vi "Periodic Tasks.vi"() -> ()   [LabVIEW 2011]
doc: "This VI runs in parallel to other tasks. It can contain as many user-defined periodic loops as you need. These can carry out PID or other sorts of timed response."
uses:
  <vilib>/Rock Robotics/SystemInterfaces/Utilities/FPGA_UtilitiesLED State.ctl
  <vilib>/Rock Robotics/SystemInterfaces/Utilities/FPGA_UtilitiesLED Source.ctl
  <vilib>/Rock Robotics/WPI/Relay/WPI_RelayValue.ctl
  Robot Global Data.vi
panel:
  out "Sent?":string="File Wrote"
  out "Voltage":dbl
  in  "Recording Array":dbl[][](array[numeric])
  in  "Turn on Record 2":bool
  out "Auton Recording 2":bool
  in  "Home Speed 2":dbl=1.0
  out "Ramp ACT Pot 2":dbl
  out "Auton Recording":bool
  in  "Turn on Record":bool
  in  "Auton Array":dbl[][](array[numeric])
  out "Right Rate":dbl
  out "Right Direction":bool
  out "Right Distance":dbl
  out "Shooter Encoder Distance":dbl
  out "Shooter Direction":bool
  out "Shooter Encoder Rate":dbl
  out "Left Rate":dbl
  out "Gyro Rate":dbl
  out "Gyro Angle":dbl
  out "Left Direction":bool
  out "Left Distance":dbl
  # "Auton Recording"
  # "Sensor Feedback"
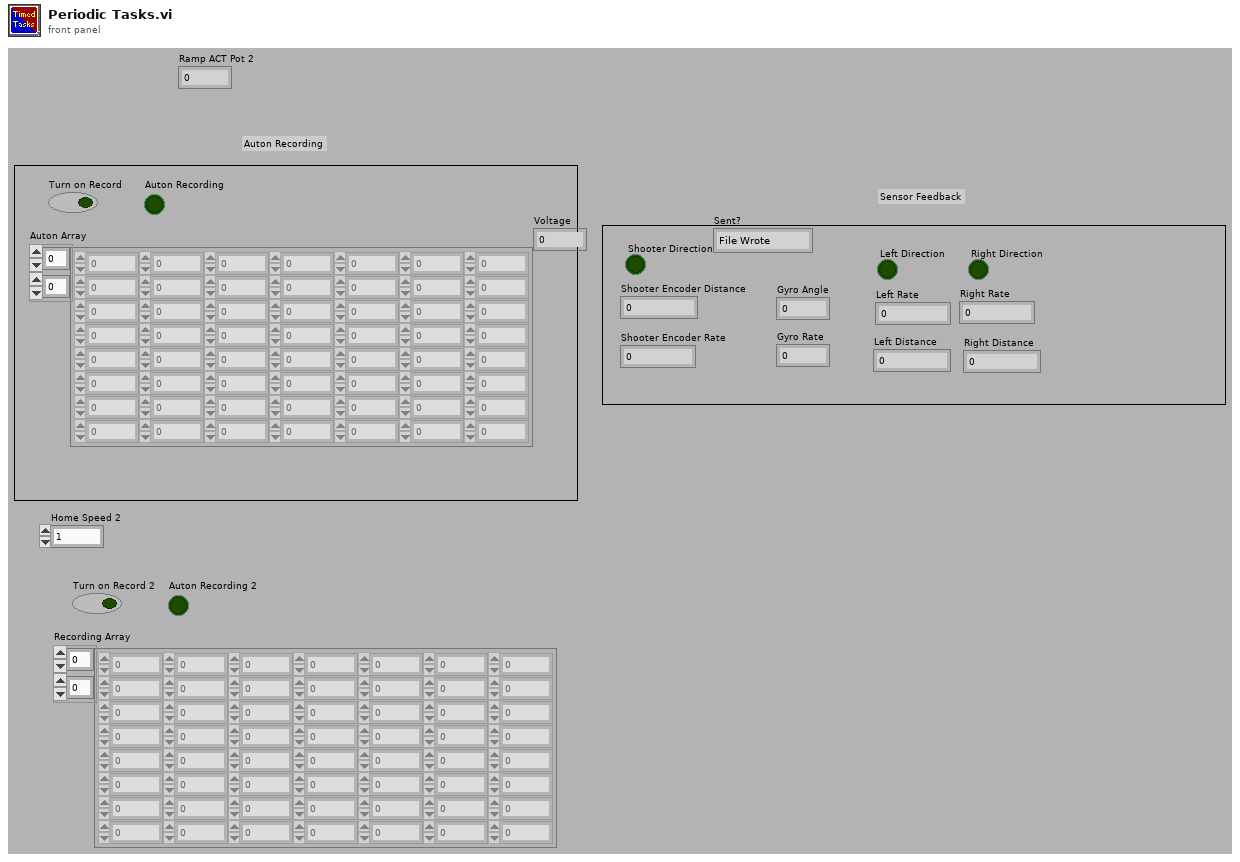
[diagram p1: front panel]
types:
  T1 = typedef "WPI_RelayValue.ctl" = enum16{"Off", "On", "Forward", "Reverse"}
  T2 = cluster{"Driver Station Digital Input (1-8)[0]":bool, "Driver Station Digital Input (1-8)[1]":bool, "Driver Station Digital Input (1-8)[2]":bool, "Driver Station Digital Input (1-8)[3]":bool, "Driver Station Digital Input (1-8)[4]":bool, "Driver Station Digital Input (1-8)[5]":bool, "Driver Station Digital Input (1-8)[6]":bool, "Driver Station Digital Input (1-8)[7]":bool, "Driver Station Digital Input (1-8)[8]":bool}
  T3 = typedef "WPI_AnalogChannelDevRef.ctl" = cluster{"DevStatus":errorcluster, "Analog Module":T4, "Analog Channel":T5}
  T4 = typedef "FPGA_TypedefAnalogModule.ctl" = enum16{"Analog Module 1", "Analog Module 2"}
  T5 = typedef "FPGA_AIChannel.ctl" = enum8{"AI 1", "AI 2", "AI 3", "AI 4", "AI 5", "AI 6", "AI 7", "AI 8", "Invalid"}
  T6 = typedef "WPI_EncoderDevRef.ctl" = cluster{"DevStatus":errorcluster, "EncoderIndex":T7, "CounterIndex":T8, "DistancePerCount":dbl, "Decoding Type":T9}
  T7 = typedef "FPGA_EncoderIdx.ctl" = enum8{"Enc 0", "Enc 1", "Enc 2", "Enc 3", "Invalid"}
  T8 = typedef "FPGA_CounterCtrSystemIndex.ctl" = enum8{"Ctr 0", "Ctr 1", "Ctr 2", "Ctr 3", "Ctr 4", "Ctr 5", "Ctr 6", "Ctr 7", "Invalid"}
  T9 = typedef "WPI_EncoderType.ctl" = enum16{"1x", "2x", "4x"}
  T10 = typedef "WPI_GyroDevRef.ctl" = cluster{"DevStatus":errorcluster, "Analog Module":T4, "Analog Channel":T5, "Offset":dbl, "Gain (VoltsPerDegree/Second)":dbl}
  T11 = typedef "WPI_RelayDevRef.ctl" = cluster{"DevStatus":errorcluster, "Relay Channel":T12, "Digital Module":T13, "Relay Direction":T14}
  T12 = typedef "FPGA_DIORelayChannel.ctl" = enum8{"Relay 1", "Relay 2", "Relay 3", "Relay 4", "Relay 5", "Relay 6", "Relay 7", "Relay 8", "Invalid"}
  T13 = typedef "FPGA_TypedefDigitalModule.ctl" = enum16{"Digital Module 1", "Digital Module 2"}
  T14 = typedef "WPI_RelayDirection.ctl" = enum16{"Both directions", "Forward only", "Reverse only"}
  T15 = typedef "FPGA_UtilitiesLED State.ctl" = enum16{"Off", "On", "Toggle"}
  T16 = typedef "FPGA_UtilitiesLED Source.ctl" = enum16{"User LED", "FPGA LED"}
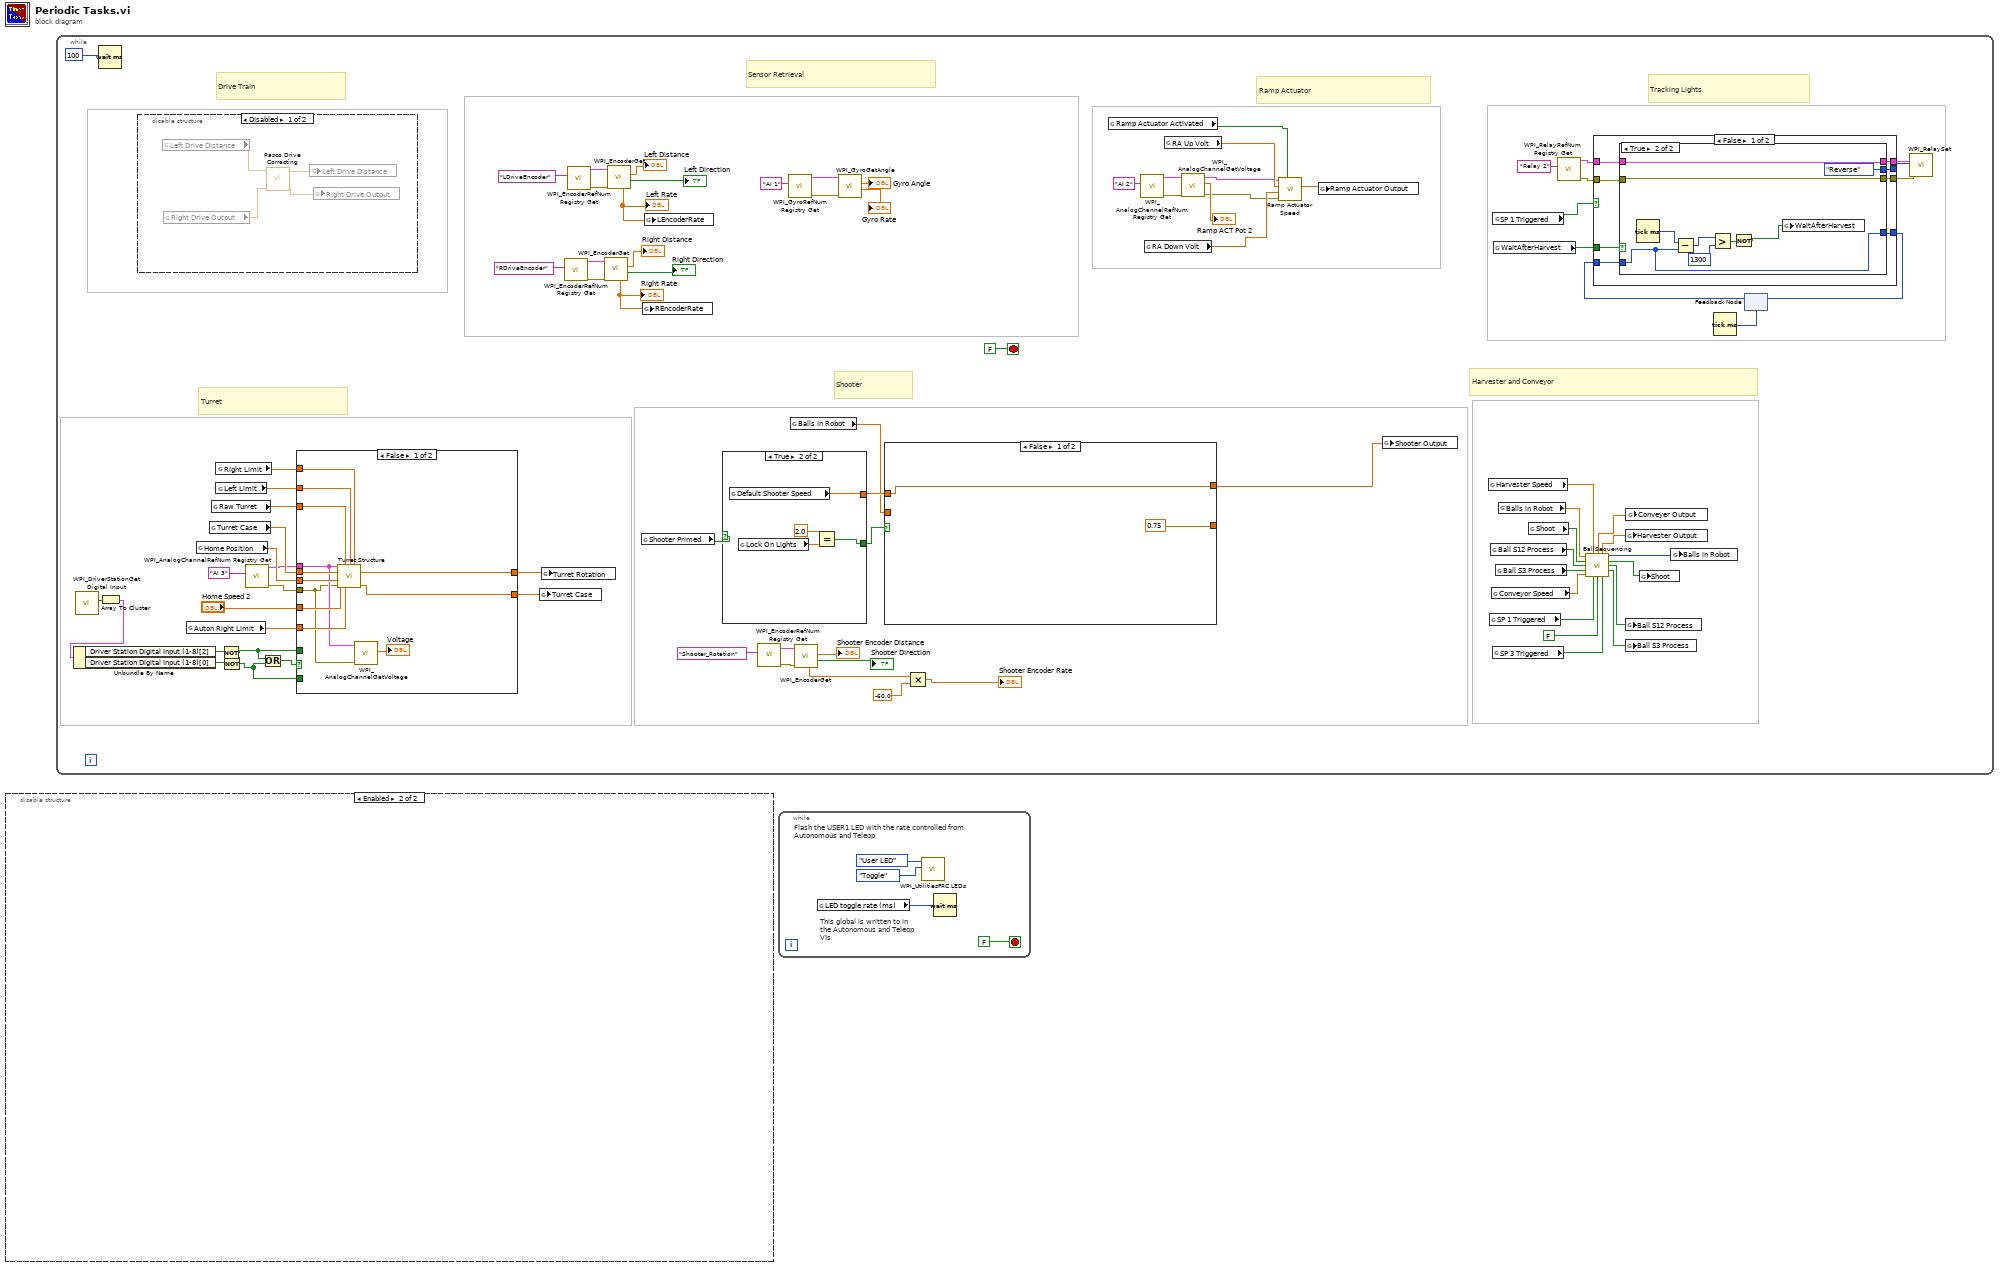
[diagram p0: block diagram]
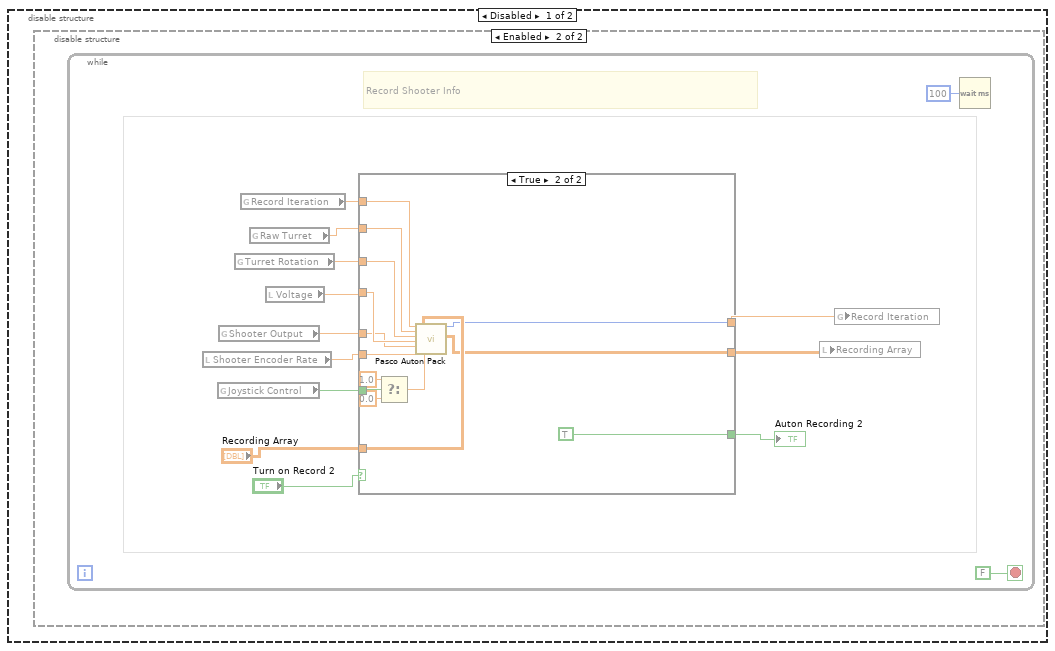
[diagram p2: hidden frame]
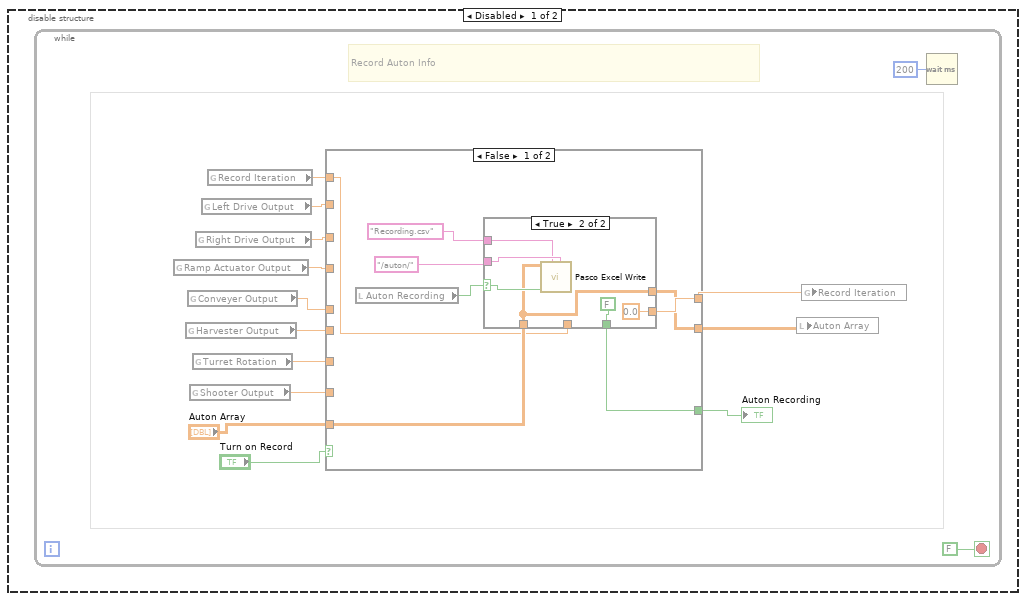
[diagram p3: hidden frame]
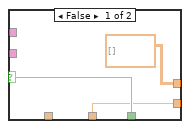
[diagram p4: hidden frame]
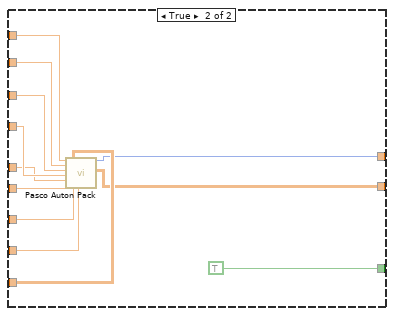
[diagram p5: hidden frame]
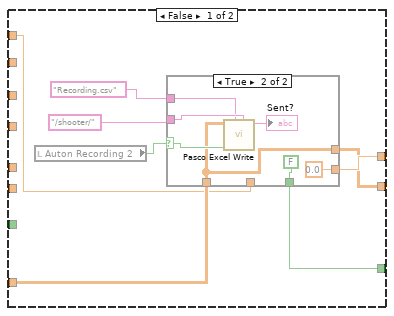
[diagram p6: hidden frame]
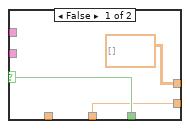
[diagram p7: hidden frame]
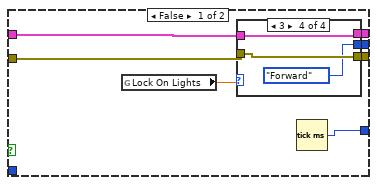
[diagram p8: hidden frame]
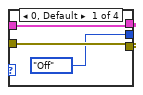
[diagram p9: hidden frame]
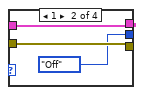
[diagram p10: hidden frame]
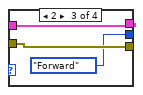
[diagram p11: hidden frame]
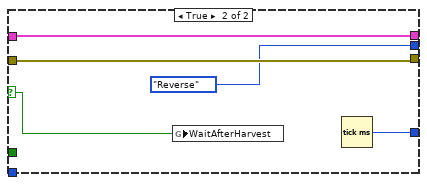
[diagram p12: hidden frame]
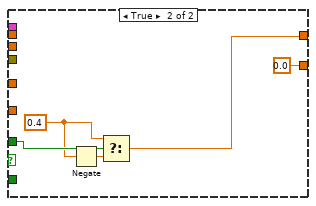
[diagram p13: hidden frame]
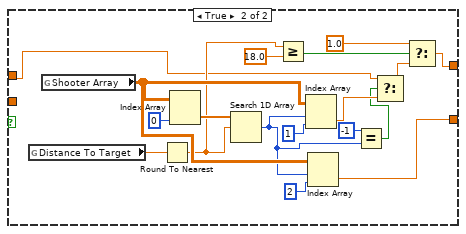
[diagram p14: hidden frame]
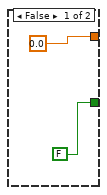
[diagram p15: hidden frame]
diagram:
  n1 = disable-structure shown="Enabled" {
    frame Disabled {
      n2 = disable-structure shown="Enabled" {
        frame Disabled {
          n3 = while {
            stop <- FALSE stop-if-true
            # "Record Auton Info"
            n4 = global read "Robot Global Data.vi" "Ramp Actuator Output"() -> (w5:dbl)
            n5 = global read "Robot Global Data.vi" "Harvester Output"() -> (w7:dbl)
            n6 = global read "Robot Global Data.vi" "Conveyer Output"() -> (w6:dbl)
            n7 = global read "Robot Global Data.vi" "Shooter Output"() -> (w9:dbl)
            n8 = global read "Robot Global Data.vi" "Turret Rotation"() -> (w8:dbl)
            n9 = global read "Robot Global Data.vi" "Right Drive Output"() -> (w4:dbl)
            n10 = global read "Robot Global Data.vi" "Left Drive Output"() -> (w3:dbl)
            n11 = global read "Robot Global Data.vi" "Record Iteration"() -> (w2:dbl)
            n12 = case shown="False" "Turn on Record" {
              tunnel: w2 -> [w19 w44]
              tunnel: w3 -> [_ w43]
              tunnel: w4 -> [_ w42]
              tunnel: w5 -> [_ w41]
              tunnel: w6 -> [_ w40]
              tunnel: w7 -> [_ w39]
              tunnel: w8 -> [_ w38]
              tunnel: w9 -> [_ w37]
              tunnel: "Auton Array" -> [w20 w36]
              tunnel: [w16 w35] -> w12
              tunnel: [w17 w34] -> w13
              tunnel: [w18 TRUE] -> w14
              frame False {
                n13 = local read "Auton Recording"() -> (w21:bool)
                n14 = case shown="True" w21 {
                  selector: w21 -> [w26 w31]
                  tunnel: [w26 FALSE] -> w18
                  tunnel: "/auton/" ("File Name") -> [_ w30]
                  tunnel: "Recording.csv" ("Folder Location") -> [_ w29]
                  tunnel: [w25 0.0 ("Record Iteration")] -> w17
                  tunnel: w19 -> [w25 _]
                  tunnel: w20 -> [_ w27]
                  tunnel: [dbl[][] [] ("Auton Array") w27] -> w16
                  frame False {
                  }
                  frame True {
                    n15 = call "Pasco Excel Write.vi"("Folder Location"=w30, "File Name"=w29, "WriteToExcel"=w31, "2D data"=w27) -> ()  [unwired: 7 in, 1 out]
                  }
                }
              }
              frame True {
                n16 = call "Pasco Auton Pack.vi"("Iterations"=w44, "Left Drive"=w43, "Right Drive"=w42, "RAMP ACT"=w41, "Conveyor"=w40, "Harvestor"=w39, "Auton Array"=w36, "Turret"=w38, "Shooter"=w37) -> ("Iteration Output"=w34:i32, "output array"=w35:dbl[][])  [unwired: 9 in]
              }
            }
            "Auton Recording" <- w14
            n17 = local write "Auton Array"(w12) -> ()
            n18 = global write "Robot Global Data.vi" "Record Iteration"(w13) -> ()
            n19 = Wait (ms)(milliseconds to wait=u32 200) -> ()  [unwired: 1 out]
          }
        }
        frame Enabled {
          n20 = while {
            stop <- FALSE stop-if-true
            # "Record Shooter Info"
            n21 = local read "Shooter Encoder Rate"() -> (w46:dbl)
            n22 = global read "Robot Global Data.vi" "Joystick Control"() -> (w45:bool)
            n23 = global read "Robot Global Data.vi" "Shooter Output"() -> (w47:dbl)
            n24 = global read "Robot Global Data.vi" "Turret Rotation"() -> (w49:dbl)
            n25 = global read "Robot Global Data.vi" "Record Iteration"() -> (w52:dbl)
            n26 = global read "Robot Global Data.vi" "Raw Turret"() -> (w50:dbl)
            n27 = local read "Voltage"() -> (w48:dbl)
            n28 = case shown="True" "Turn on Record 2" {
              tunnel: w52 -> [w62 w90]
              tunnel: w50 -> [_ w89]
              tunnel: w49 -> [_ w88]
              tunnel: w48 -> [_ w87]
              tunnel: w47 -> [_ w86]
              tunnel: w46 -> [_ w85]
              tunnel: "Recording Array" -> [w63 w84]
              tunnel: [w59 w83] -> w55
              tunnel: [w60 w82] -> w56
              tunnel: [w61 TRUE] -> w57
              tunnel: w45 -> [_ w80]
              frame False {
                n29 = local read "Auton Recording 2"() -> (w64:bool)
                n30 = case shown="True" w64 {
                  selector: w64 -> [w69 w75]
                  tunnel: [w69 FALSE] -> w61
                  tunnel: "/shooter/" ("File Name") -> [_ w74]
                  tunnel: "Recording.csv" ("Folder Location") -> [_ w73]
                  tunnel: [w68 0.0 ("Record Iteration")] -> w60
                  tunnel: w62 -> [w68 _]
                  tunnel: w63 -> [_ w71]
                  tunnel: [dbl[][] [] ("Auton Array") w71] -> w59
                  frame False {
                  }
                  frame True {
                    n31 = call "Pasco Excel Write.vi"("Folder Location"=w74, "File Name"=w73, "WriteToExcel"=w75, "2D data"=w71) -> ("Sent?"=→"Sent?":string)  [unwired: 7 in]
                  }
                }
              }
              frame True {
                n32 = Select(t=1.0, s=w80, f=0.0) -> (s? t:f=w77:dbl)
                n33 = call "Pasco Auton Pack.vi"("Iterations"=w90, "Left Drive"=w89, "Right Drive"=w88, "RAMP ACT"=w87, "Conveyor"=w86, "Harvestor"=w85, "Auton Array"=w84, "Turret"=w77) -> ("Iteration Output"=w82:i32, "output array"=w83:dbl[][])  [unwired: 10 in]
              }
            }
            "Auton Recording 2" <- w57
            n34 = local write "Recording Array"(w55) -> ()
            n35 = global write "Robot Global Data.vi" "Record Iteration"(w56) -> ()
            n36 = Wait (ms)(milliseconds to wait=u32 100) -> ()  [unwired: 1 out]
          }
        }
      }
    }
    frame Enabled {
    }
  }
  n37 = while {
    stop <- FALSE stop-if-true
    # "Tracking Lights"
    # "Harvester and Conveyor"
    # "Shooter"
    # "Sensor Retrieval"
    # "Turret"
    # "Drive Train"
    # "Ramp Actuator"
    n38 = call <vilib>:"WPI_DriverStationGet Digital Input.vi"() -> ("Driver Station Digital Input (1-8)"=w120:bool[])  [unwired: 11 in]
    n39 = Wait (ms)(milliseconds to wait=u32 100) -> ()  [unwired: 1 out]
    n40 = Array To Cluster(array=w120) -> (cluster=w119:T2)
    n41 = Unbundle By Name(w119) -> ("Driver Station Digital Input (1-8)[2]"=w105:bool, "Driver Station Digital Input (1-8)[0]"=w103:bool)
    n42 = disable-structure shown="Disabled" {
      frame Disabled {
        n43 = global read "Robot Global Data.vi" "Left Drive Distance"() -> (w265:dbl)
        n44 = global read "Robot Global Data.vi" "Right Drive Output"() -> (w264:dbl)
        n45 = call "Pasco Drive Correcting.vi"("RightDriveOutput"=w264, "LeftDriveOutput"=w265) -> ("RightDriveOutput"=w262:dbl, "LeftDriveOutput"=w263:dbl)  [unwired: 8 in]
        n46 = global write "Robot Global Data.vi" "Left Drive Distance"(w263) -> ()
        n47 = global write "Robot Global Data.vi" "Right Drive Output"(w262) -> ()
      }
      frame Enabled {
      }
    }
    n48 = global read "Robot Global Data.vi" "Auton Right Limit"() -> (w116:dbl)
    n49 = global read "Robot Global Data.vi" "Home Position"() -> (w111:dbl)
    n50 = global read "Robot Global Data.vi" "Turret Case"() -> (w110:dbl)
    n51 = global read "Robot Global Data.vi" "Raw Turret"() -> (w112:dbl)
    n52 = global read "Robot Global Data.vi" "Right Limit"() -> (w115:dbl)
    n53 = global read "Robot Global Data.vi" "Left Limit"() -> (w114:dbl)
    n54 = Not(x=w105) -> (.not. x?=w104:bool)
    n55 = Not(x=w103) -> (.not. x?=w102:bool)
    n56 = call <vilib>:"WPI_AnalogChannelRefNum Registry Get.vi"("refnum name"="AI 3") -> ("error out"=w109:errorcluster, "AIDeviceRef"=w108:T3)  [unwired: 9 in]
    n57 = Or(x=w104, y=w102) -> (x .or. y?=w106:bool)
    n58 = case shown="False" w106 {
      tunnel: w108 -> [w221 _]
      tunnel: w109 -> [w220 _]
      tunnel: w110 -> [w230 _]
      tunnel: w111 -> [w229 _]
      tunnel: w112 -> [w228 _]
      tunnel: "Home Speed 2" -> [w227 _]
      tunnel: w114 -> [w226 _]
      tunnel: w115 -> [w225 _]
      tunnel: w116 -> [w224 _]
      tunnel: [w223 w234] -> w117
      tunnel: [w222 0.0 ("Turret Case Output")] -> w118
      tunnel: w104 -> [_ w235]
      tunnel: w102 -> [_ _]
      frame False {
        n59 = call "Turret Structure.vi"("AIDeviceRef"=w221, "Raw Turret"=w228, "Left"=w226, "Right"=w225, "Turret Case"=w230, "Home Speed"=w227, "Home postion"=w229, "error in (no error)"=w220, "Auton Right"=w224) -> ("Turret Output"=w223:dbl, "Turret Case Output"=w222:dbl)  [unwired: 5 in]
        n60 = call <vilib>:"WPI_AnalogChannelGetVoltage.vi"("error in (no error)"=w220, "AIDeviceRef"=w221) -> ("Voltage"=→"Voltage":dbl)  [unwired: 7 in, 2 out]
      }
      frame True {
        w231 = 0.4 ("t")
        n61 = Negate(x=w231) -> (-x=w232:dbl)
        n62 = Select(t=w231, s=w235, f=w232) -> (s? t:f=w234:dbl)
      }
    }
    n63 = global write "Robot Global Data.vi" "Turret Case"(w118) -> ()
    n64 = global write "Robot Global Data.vi" "Turret Rotation"(w117) -> ()
    n65 = call <vilib>:"WPI_EncoderRefNum Registry Get.vi"("refnum name"="RDriveEncoder") -> ("error out"=w144:errorcluster, "EncoderDevRef"=w143:T6)  [unwired: 9 in]
    n66 = call <vilib>:"WPI_EncoderRefNum Registry Get.vi"("refnum name"="LDriveEncoder") -> ("error out"=w150:errorcluster, "EncoderDevRef"=w149:T6)  [unwired: 9 in]
    n67 = call <vilib>:"WPI_EncoderGet.vi"("error in (no error)"=w144, "EncoderDevRef"=w143) -> ("Direction"=→"Right Direction":bool, "Distance"=→"Right Distance":dbl, "Rate"=w140:dbl)  [unwired: 4 in, 3 out]
    "Right Rate" <- w140
    n68 = call <vilib>:"WPI_EncoderGet.vi"("error in (no error)"=w150, "EncoderDevRef"=w149) -> ("Direction"=→"Left Direction":bool, "Distance"=→"Left Distance":dbl, "Rate"=w146:dbl)  [unwired: 4 in, 3 out]
    "Left Rate" <- w146
    n69 = global read "Robot Global Data.vi" "Shooter Primed"() -> (w164:bool)
    n70 = global write "Robot Global Data.vi" "REncoderRate"(w140) -> ()
    n71 = global write "Robot Global Data.vi" "LEncoderRate"(w146) -> ()
    n72 = case shown="True" w164 {
      tunnel: [FALSE ("Shooter Primed") w258] -> w122
      tunnel: [0.0 w259] -> w162
      frame False {
      }
      frame True {
        n73 = global read "Robot Global Data.vi" "Default Shooter Speed"() -> (w259:dbl)
        n74 = global read "Robot Global Data.vi" "Lock On Lights"() -> (w261:dbl)
        n75 = Equal?(x=2.0, y=w261) -> (x = y?=w258:bool)
      }
    }
    n76 = call <vilib>:"WPI_EncoderRefNum Registry Get.vi"("refnum name"="Shooter_Rotation") -> ("error out"=w124:errorcluster, "EncoderDevRef"=w125:T6)  [unwired: 9 in]
    n77 = call <vilib>:"WPI_GyroRefNum Registry Get.vi"("refnum name"="AI 1") -> ("error out"=w158:errorcluster, "GyroDevRef"=w159:T10)  [unwired: 9 in]
    n78 = global read "Robot Global Data.vi" "Balls in Robot"() -> (w161:dbl)
    n79 = call <vilib>:"WPI_EncoderGet.vi"("error in (no error)"=w124, "EncoderDevRef"=w125) -> ("Direction"=→"Shooter Direction":bool, "Distance"=→"Shooter Encoder Distance":dbl, "Rate"=w121:dbl)  [unwired: 4 in, 3 out]
    n80 = call <vilib>:"WPI_GyroGetAngle.vi"("error in (no error)"=w158, "GyroDevRef"=w159) -> ("Angular Rate"=→"Gyro Rate":dbl, "Angle"=→"Gyro Angle":dbl)  [unwired: 6 in, 2 out]
    n81 = case shown="False" w122 {
      tunnel: [w237 w246] -> w163
      tunnel: w162 -> [w237 w238]
      tunnel: w161 -> [_ _]
      tunnel: [0.75 w255] -> _
      frame False {
      }
      frame True {
        n82 = global read "Robot Global Data.vi" "Distance To Target"() -> (w252:dbl)
        n83 = global read "Robot Global Data.vi" "Shooter Array"() -> (w249:dbl[][])
        n84 = Round To Nearest(number=w252) -> (nearest integer value=w247:dbl)
        n85 = Index Array(array=w249, index (col)=0 ("disabled index (col)")) -> (element=w251:dbl[])  [unwired: 1 in]
        n86 = Search 1D Array(1D array=w251, element=w247) -> (index of element=w241:i32)  [unwired: 1 in]
        n87 = Greater Or Equal?(x=w247, y=18.0) -> (x >= y?=w245:bool)
        n88 = Index Array(array=w249, index (row)=w241, index (col)=1 ("disabled index (col)")) -> (element=w242:dbl)
        n89 = Index Array(array=w249, index (row)=w241, index (col)=2 ("disabled index (col)")) -> (element=w255:dbl)
        n90 = Equal?(x=-1, y=w241) -> (x = y?=w239:bool)
        n91 = Select(t=w238, s=w239, f=w242) -> (s? t:f=w243:dbl)
        n92 = Select(t=1.0, s=w245, f=w243) -> (s? t:f=w246:dbl)
      }
    }
    n93 = Multiply(x=w121, y=-60.0) -> (x*y=→"Shooter Encoder Rate":dbl)
    n94 = global read "Robot Global Data.vi" "Ramp Actuator Activated"() -> (w135:bool)
    n95 = call <vilib>:"WPI_AnalogChannelRefNum Registry Get.vi"("refnum name"="AI 2") -> ("error out"=w133:errorcluster, "AIDeviceRef"=w134:T3)  [unwired: 9 in]
    n96 = global read "Robot Global Data.vi" "RA Down Volt"() -> (w138:dbl)
    n97 = global read "Robot Global Data.vi" "RA Up Volt"() -> (w137:dbl)
    n98 = call <vilib>:"WPI_AnalogChannelGetVoltage.vi"("error in (no error)"=w133, "AIDeviceRef"=w134) -> ("error out"=w130:errorcluster, "Voltage"=→"Ramp ACT Pot 2":dbl, "AIDeviceRef"=w131:T3)  [unwired: 7 in]
    n99 = call "Ramp Actuator Speed.vi"("Up to Down"=w135, "error in (no error)"=w130, "RA Down Volt"=w138, "RA Up Volt"=w137, "AIDeviceRef"=w131) -> ("Ramp Actuator Ouput"=w136:dbl)  [unwired: 6 in]
    n100 = global write "Robot Global Data.vi" "Ramp Actuator Output"(w136) -> ()
    n101 = global write "Robot Global Data.vi" "Shooter Output"(w163) -> ()
    n102 = global read "Robot Global Data.vi" "Harvester Speed"() -> (w160:dbl)
    n103 = global read "Robot Global Data.vi" "SP 1 Triggered"() -> (w167:bool)
    n104 = global read "Robot Global Data.vi" "Ball S12 Process"() -> (w169:bool)
    n105 = global read "Robot Global Data.vi" "Conveyor Speed"() -> (w152:dbl)
    n106 = global read "Robot Global Data.vi" "SP 3 Triggered"() -> (w166:bool)
    n107 = global read "Robot Global Data.vi" "SP 1 Triggered"() -> (w101:bool)
    n108 = global read "Robot Global Data.vi" "WaitAfterHarvest"() -> (w94:bool)
    n109 = global read "Robot Global Data.vi" "Ball S3 Process"() -> (w168:bool)
    n110 = global read "Robot Global Data.vi" "Balls in Robot"() -> (w171:dbl)
    n111 = global read "Robot Global Data.vi" "Shoot"() -> (w170:bool)
    n112 = call <vilib>:"WPI_RelayRefNum Registry Get.vi"("refnum name"="Relay 2") -> ("error out"=w99:errorcluster, "RelayDevRef"=w97:T11)  [unwired: 9 in]
    n113 = call "BallSequencing.vi"("Balls In Robot"=w171, "Speed of Harvester"=w160, "Shoot"=w170, "Ball S12 Process"=w169, "Ball S3 Process"=w168, "Speed of Conveyor"=w152, "SP 1 Triggered"=w167, "SP 2 Triggered"=FALSE, "SP 3 Triggered"=w166) -> ("Conveyer Output"=w172:dbl, "Harvester Output"=w173:dbl, "Balls In Robot Output"=w154:i32, "Shoot Output"=w153:bool, "Ball S12 Process Output"=w175:bool, "Ball S3 Process Output"=w174:bool)  [unwired: 1 in]
    n114 = global write "Robot Global Data.vi" "Harvester Output"(w173) -> ()
    n115 = global write "Robot Global Data.vi" "Ball S12 Process"(w175) -> ()
    n116 = global write "Robot Global Data.vi" "Ball S3 Process"(w174) -> ()
    n117 = global write "Robot Global Data.vi" "Conveyer Output"(w172) -> ()
    n118 = global write "Robot Global Data.vi" "Shoot"(w153) -> ()
    n119 = global write "Robot Global Data.vi" "Balls in Robot"(w154) -> ()
    n120 = Tick Count (ms)() -> (millisecond timer value=w91:u32)
    n121 = feedback #1(w91) -> (w92:u32)
    n122 = case shown="False" w101 {
      selector: w101 -> [_ w215]
      tunnel: [w185 w218] -> w96
      tunnel: w97 -> [w184 w218]
      tunnel: [w183 w217] -> w98
      tunnel: w99 -> [w182 w217]
      tunnel: [w181 WPI_RelayValue."Reverse" ("RelayValue")] -> w100
      tunnel: [w178 w214] -> w93
      tunnel: w94 -> [w180 _]
      tunnel: w92 -> [w179 _]
      frame False {
        n123 = case shown="True" w180 {
          tunnel: [w192 w213] -> w185
          tunnel: w184 -> [w191 w213]
          tunnel: [w190 w212] -> w183
          tunnel: w182 -> [w189 w212]
          tunnel: [w188 WPI_RelayValue."Reverse" ("RelayValue")] -> w181
          tunnel: w179 -> [_ w205]
          tunnel: [w186 w205] -> w178
          frame False {
            n124 = global read "Robot Global Data.vi" "Lock On Lights"() -> (w187:dbl)
            n125 = case shown="3" w187 {
              tunnel: [w195 w198 w201 w204] -> w192
              tunnel: w191 -> [w195 w198 w201 w204]
              tunnel: [w194 w197 w200 w203] -> w190
              tunnel: w189 -> [w194 w197 w200 w203]
              tunnel: [WPI_RelayValue."Off" ("RelayValue") WPI_RelayValue."Off" ("RelayValue") WPI_RelayValue."Forward" ("RelayValue") WPI_RelayValue."Forward" ("RelayValue")] -> w188
              frame 0, Default {
              }
              frame 1 {
              }
              frame 2 {
              }
              frame 3 {
              }
            }
            n126 = Tick Count (ms)() -> (millisecond timer value=w186:u32)
          }
          frame True {
            n127 = Tick Count (ms)() -> (millisecond timer value=w210:u32)
            n128 = Subtract(x=w210, y=w205) -> (x-y=w209:u32)
            n129 = Greater?(x=w209, y=u32 1300) -> (0:w207:bool)
            n130 = Not(x=w207) -> (.not. x?=w206:bool)
            n131 = global write "Robot Global Data.vi" "WaitAfterHarvest"(w206) -> ()
          }
        }
      }
      frame True {
        n132 = global write "Robot Global Data.vi" "WaitAfterHarvest"(w215) -> ()
        n133 = Tick Count (ms)() -> (millisecond timer value=w214:u32)
      }
    }
    n134 = feedback-in #1(w93) -> ()
    n135 = call <vilib>:"WPI_RelaySet.vi"("error in (no error)"=w98, "RelayValue"=w100, "RelayDevRef"=w96) -> ()  [unwired: 7 in, 2 out]
  }
  n136 = while {
    stop <- FALSE stop-if-true
    # "This global is written to in the Autonomous and Teleop VIs"
    # "Flash the USER1 LED with the rate controlled from Autonomous and Teleop"
    n137 = global read "Robot Global Data.vi" "LED toggle rate (ms)"() -> (w266:u32)
    n138 = call <vilib>:"WPI_UtilitiesFRC LEDs.vi"("State"=FPGA_UtilitiesLED_State."Toggle", "LED Type"=FPGA_UtilitiesLED_Source."User LED") -> ()  [unwired: 1 in, 9 out]
    n139 = Wait (ms)(milliseconds to wait=w266) -> ()  [unwired: 1 out]
  }
